vi "addDataBooleanArray.vi"(8 "error in (no error)":errorcluster, 9 "Length":i32, 10 "Data":bool[](array[boolean]), 11 "U8ArrayBuilderAutoIndexing in":refnum<class "U8ArrayBuilderAutoIndexing.lvclass">) -> (0 "error out":errorcluster, 3 "U8ArrayBuilderAutoIndexing out":refnum<class "U8ArrayBuilderAutoIndexing.lvclass">)   [LabVIEW 2016, in "RTUtilities.lvlib" / "U8ArrayBuilderAutoIndexing.lvclass"]
uses:
  U8ArrayBuilderAutoIndexing.lvclass
  U8ArrayBuilderAutoIndexing.lvclass/U8ArrayBuilderAutoIndexing.ctl
  U8ArrayBuilderManualIndexing/U8ArrayBuilderManualIndexing.lvclass
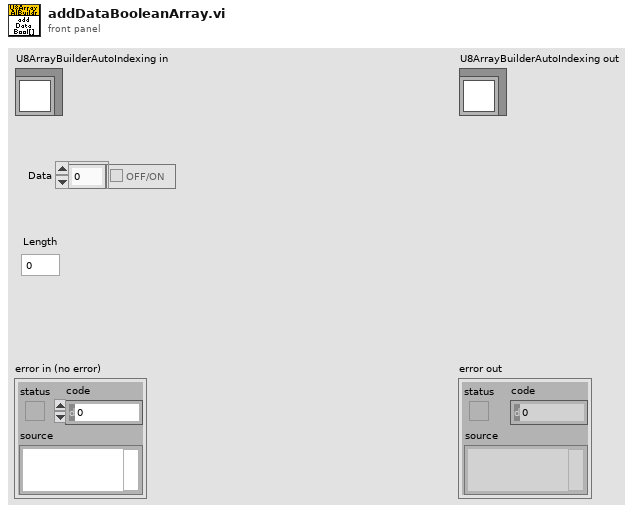
[diagram p1: front panel]
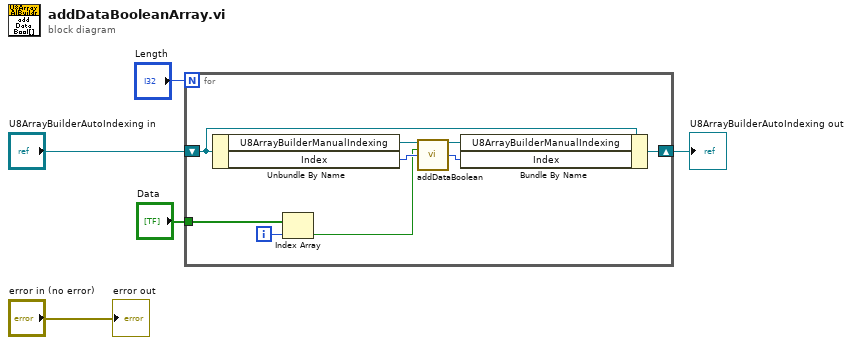
[diagram p0: block diagram]
diagram:
  n1 = for {
    N: "Length" -> [_]
    shift-right: [w13] -> w3
    shift-left: "U8ArrayBuilderAutoIndexing in" -> [w14]
    tunnel: "Data" -> [w8]
    i -> [w7]
    n2 = Unbundle By Name(w14) -> ("U8ArrayBuilderManualIndexing"=w12:refnum<class "U8ArrayBuilderManualIndexing.lvclass">, "Index"=w11:i32)
    n3 = Index Array(array=w8, index=w7) -> (element=w6:bool)
    n4 = call "addDataBoolean.vi"("U8ArrayBuilderManualIndexing in"=w12, "Data"=w6, "Index"=w11) -> ("U8ArrayBuilderManualIndexing out"=w9:refnum<class "U8ArrayBuilderManualIndexing.lvclass">, "Index out"=w10:i32)  [unwired: 10 in, 1 out]
    n5 = Bundle By Name(cluster=w14, "U8ArrayBuilderManualIndexing"=w9, "Index"=w10) -> (w13:refnum<class "U8ArrayBuilderAutoIndexing.lvclass">)
  }
  "U8ArrayBuilderAutoIndexing out" <- w3
  "error out" <- "error in (no error)"
